vi "ExposeRemoveParameter.vi"(9 "Parameter":variant, 10 "Name":string, 11 "Expose Info":T1) -> ()   [LabVIEW 2017]
uses:
  Core/ExposeInfo.ctl
  C:/Code/CMCryoSysCode/Expose/COM/CSCom/CSCom/bin/Release/CSCom.dll
  COM/CSCom/CSCom/bin/Release/CSCom.dll
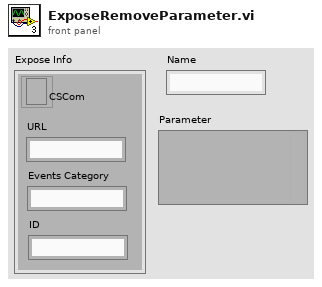
[diagram p1: front panel]
types:
  T1 = typedef "ExposeInfo.ctl" = cluster{"CSCom":refnum<k24>, "URL":string, "Events Category":string, "ID":string}
  T2 = typedef "ExposeDataType.ctl" = cluster{"Values":variant, "ParameterBindingInfo":variant}
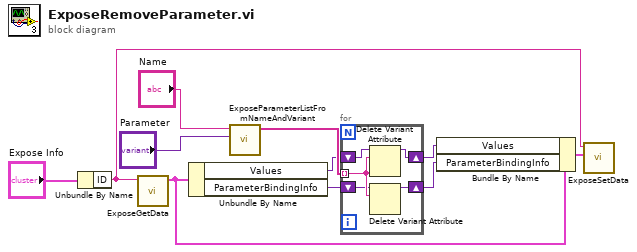
[diagram p0: block diagram]
diagram:
  n1 = Unbundle By Name("Expose Info") -> ("ID"=w10:string)
  n2 = call "ExposeGetData.vi"("ExposeID"=w10) -> ("ExposeDataType"=w4:T2)  [unwired: 9 in, 1 out]
  n3 = Unbundle By Name(w4) -> ("Values"=w6:variant, "ParameterBindingInfo"=w5:variant)
  n4 = call "ExposeParameterListFromNameAndVariant.vi"("Parameter"="Parameter", "Name (empty)"="Name") -> ("Parameter names"=w7:string[])  [unwired: 8 in, 1 out]
  n5 = for {
    tunnel: w7 -> [w14] mode=indexing
    shift-right: [w15] -> w3
    shift-left: w6 -> [w16]
    shift-right: [w12] -> w2
    shift-left: w5 -> [w13]
    n6 = Delete Variant Attribute(6:w14, 7:w16) -> (3:w15:variant)  [unwired: 1 in, 2 out]
    n7 = Delete Variant Attribute(6:w14, 7:w13) -> (3:w12:variant)  [unwired: 1 in, 2 out]
  }
  n8 = Bundle By Name(cluster=w4, "Values"=w3, "ParameterBindingInfo"=w2) -> (w1:T2)
  n9 = call "ExposeSetData.vi"("ExposeDataType"=w1, "ExposeID"=w10) -> ()  [unwired: 10 in]
